vi "CreatePinmapWith3Pins_QueryPins_3PinsReported.vi"() -> (6 "pass":bool, 8 "result":string, 15 "error out":errorcluster)   [LabVIEW 2020]
uses:
  Runtime/MeasurementLink Pin Map Client/RPC Messages/ni_measurementlink_pinmap_v1_CreatePinMapFromXmlRequest.ctl
  Runtime/MeasurementLink Pin Map Client/RPC Messages/ni_measurementlink_pinmap_v1_QueryPinsRequest.ctl
  Runtime/MeasurementLink Pin Map Client/RPC Messages/ni_measurementlink_pinmap_v1_PinDefinition.ctl
  65b5dcd1-a9b7-4222-a274-75e5d4c706a6.vi
  e379b5ff-d65c-4c10-92db-bffab39ca4f8.vi
  <vilib>/Comparison/Less/Less Functor/Less Functor.lvclass
  Runtime/MeasurementLink Pin Map Client/MeasurementLink Pin Map Client.lvlib
  Runtime/MeasurementLink Discovery V1/MeasurementLink Discovery V1.lvlib
panel:
  # "Test assumes discovery service and pin map service have already been started."
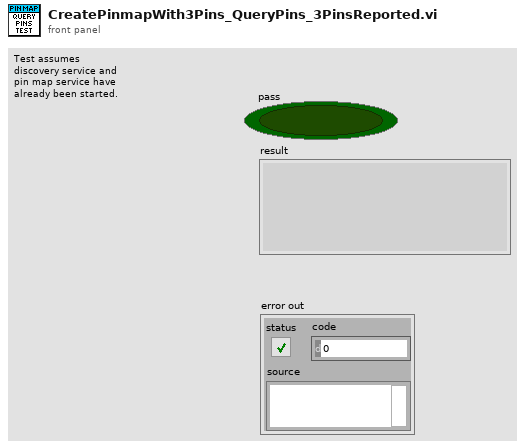
[diagram p1: front panel]
types:
  T1 = typedef "MeasurementLink Pin Map Client.lvlib/ni_measurementlink_pinmap_v1_PinDefinition.ctl" = cluster{"display_name":string, "is_system_pin":bool}
  T2 = typedef "MeasurementLink Pin Map Client.lvlib/ni_measurementlink_pinmap_v1_QueryPinsRequest.ctl" = cluster{"pin_map_id":string, "instrument_type_id":string}
  T3 = typedef "MeasurementLink Pin Map Client.lvlib/ni_measurementlink_pinmap_v1_CreatePinMapFromXmlRequest.ctl" = cluster{"pin_map_id":string, "pin_map_xml":string}
  T4 = typedef "grpc-lvsupport-release.lvlib/grpcId.ctl" = u64
  T5 = typedef "MeasurementLink Pin Map Client.lvlib/ni_measurementlink_pinmap_v1_PinMap.ctl" = cluster{"pin_map_id":string}
  T6 = typedef "MeasurementLink Pin Map Client.lvlib/ni_measurementlink_pinmap_v1_QueryPinsResponse.ctl" = cluster{"pins":T1[], "pin_groups":T7[]}
  T7 = typedef "MeasurementLink Pin Map Client.lvlib/ni_measurementlink_pinmap_v1_PinGroupDefinition.ctl" = cluster{"display_name":string, "pin_or_group_references":string[], "resolved_pins":string[]}
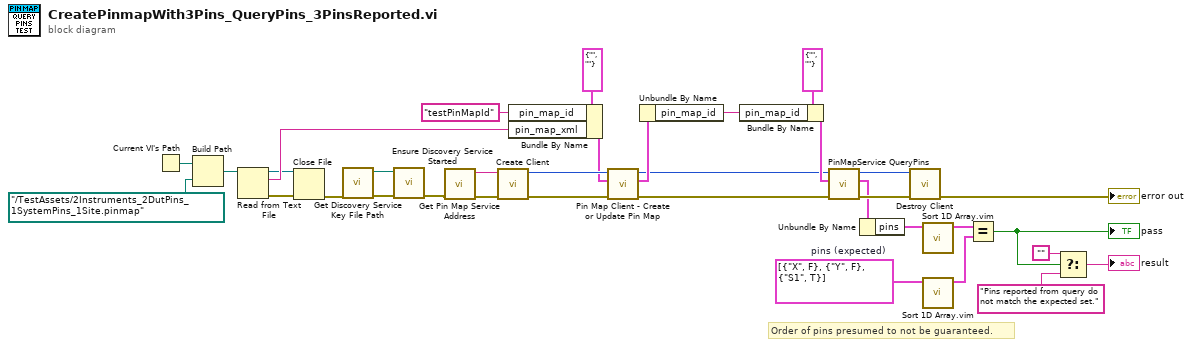
[diagram p0: block diagram]
diagram:
  w5 = T1[] [{"display_name"="X", "is_system_pin"=FALSE}, {"display_name"="Y", "is_system_pin"=FALSE}, {"display_name"="S1", "is_system_pin"=TRUE}]  # pins (expected)
  # "Order of pins presumed to not be guaranteed."
  n1 = Current VI's Path() -> (path=w33:path)
  n2 = Build Path(base path=w33, name or relative path=path "../TestAssets/2Instruments_2DutPins_1SystemPins_1Site.pinmap") -> (appended path=w31:path)
  n3 = Read from Text File(file (use dialog)=w31) -> (refnum out=w27:refnum<file>, text=w29:string, error out=w28:errorcluster)  [unwired: 3 in, 1 out]
  n4 = Close File(refnum=w27, error in=w28) -> (error out=w2:errorcluster)  [unwired: 1 out]
  n5 = call "Get Discovery Service Key File Path.vi"("error in"=w2) -> ("error out"=w4:errorcluster, "key file path"=w3:path)  [unwired: 9 in]
  n6 = call "Ensure Discovery Service Started.vi"("error in"=w4, "path"=w3) -> ("error out"=w1:errorcluster)  [unwired: 8 in, 1 out]
  n7 = call "Get Pin Map Service Address.vi"("error in (no error)"=w1) -> ("error out"=w18:errorcluster, "address"=w19:string)  [unwired: 9 in]
  n8 = call "Create Client.vi"("error in"=w18, "address"=w19) -> ("error out"=w34:errorcluster, "gRPC ID Out"=w9:T4)  [unwired: 8 in]
  n9 = Bundle By Name(cluster=T3 {"pin_map_id"="", "pin_map_xml"=""} ("Request Data"), "pin_map_id"="testPinMapId", "pin_map_xml"=w29) -> (w8:T3)
  n10 = call "Pin Map Client - Create or Update Pin Map.vi"("error in (no error)"=w34, "Request Data"=w8, "gRPC ID Out"=w9) -> ("error out"=w26:errorcluster, "Response Data"=w7:T5, "gRPC ID out"=w6:T4)  [unwired: 6 in]
  n11 = Unbundle By Name(w7) -> ("pin_map_id"=w22:string)
  n12 = Bundle By Name(cluster=T2 {"pin_map_id"="", "instrument_type_id"=""} ("Request Data"), "pin_map_id"=w22) -> (w21:T2)
  n13 = call "PinMapService QueryPins.vi"("error in"=w26, "Request Data"=w21, "gRPC ID"=w6) -> ("error out"=w25:errorcluster, "Response Data"=w20:T6, "gRPC ID out"=w24:T4)  [unwired: 6 in]
  n14 = Unbundle By Name(w20) -> ("pins"=w17:T1[])
  n15 = call "Destroy Client.vi"("error in"=w25, "gRPC ID"=w24) -> ("error out"=→"error out":errorcluster)  [unwired: 9 in]
  n16 = call "Sort 1D Array.vim"("unsorted array"=w17) -> ("sorted array"=w16:T1[])  [unwired: 10 in]
  n17 = call "Sort 1D Array.vim"("unsorted array"=w5) -> ("sorted array"=w15:T1[])  [unwired: 10 in]
  n18 = Equal?(x=w16, y=w15) -> (x = y?=w14:bool)
  "pass" <- w14
  n19 = Select(t="", s=w14, f="Pins reported from query do not match the expected set." ("display_name")) -> (s? t:f=→"result":string)
